vi "ValidateConfig.vi"(8 "error in (no error)":errorcluster, 11 "Channel in":refnum<class "Channel.lvclass">) -> (0 "error out":errorcluster, 2 "valid?":bool, 3 "Channel out":refnum<class "Channel.lvclass">)   [LabVIEW 2018, in "Channel.lvclass"]
uses:
  Channel.lvclass
  Channel.lvclass/Channel.ctl
  Interface/Interface.lvclass/Interface.ctl
  Interface/Interface.lvclass
panel:
  # "T=valid\nF=error"
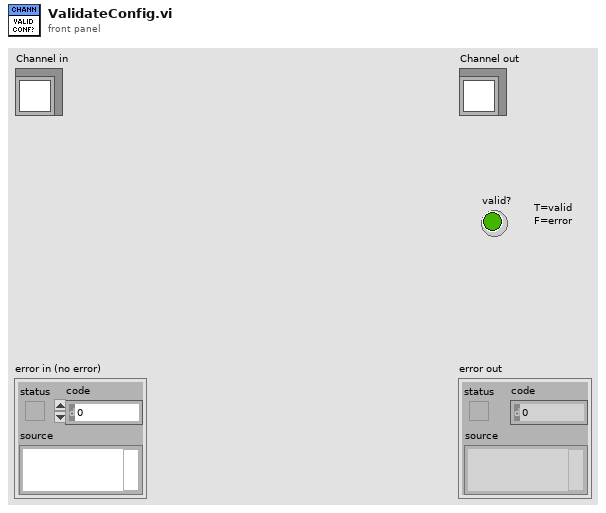
[diagram p1: front panel]
types:
  T1 = cluster{"ACQUISITION_MODE":u8, "TRIGGER_MODE":u8, "READ_MODE":u8, "PREAMP":u8, "READOUT_RATE":u8, "VERTICAL_SHIFT_SPEED":u8, "EM_MODE":u8, "EM_GAIN":u16, "SHUTTER_MODE":u8, "SHUTTER_TTL":u8, "SHUTTER_OPENING_TIME":u16, "SHUTTER_CLOSING_TIME":u16, "VBIN":u16, "HBIN":u16, "INITIAL_LINE":u16, "INITIAL_COLUMN":u16, "FINAL_LINE":u16, "FINAL_COLUMN":u16, "FRAME_TRANSFER":bool, "VERTICAL_CLOCK_VOLTAGE":u8, "AD_CHANNEL":u32}
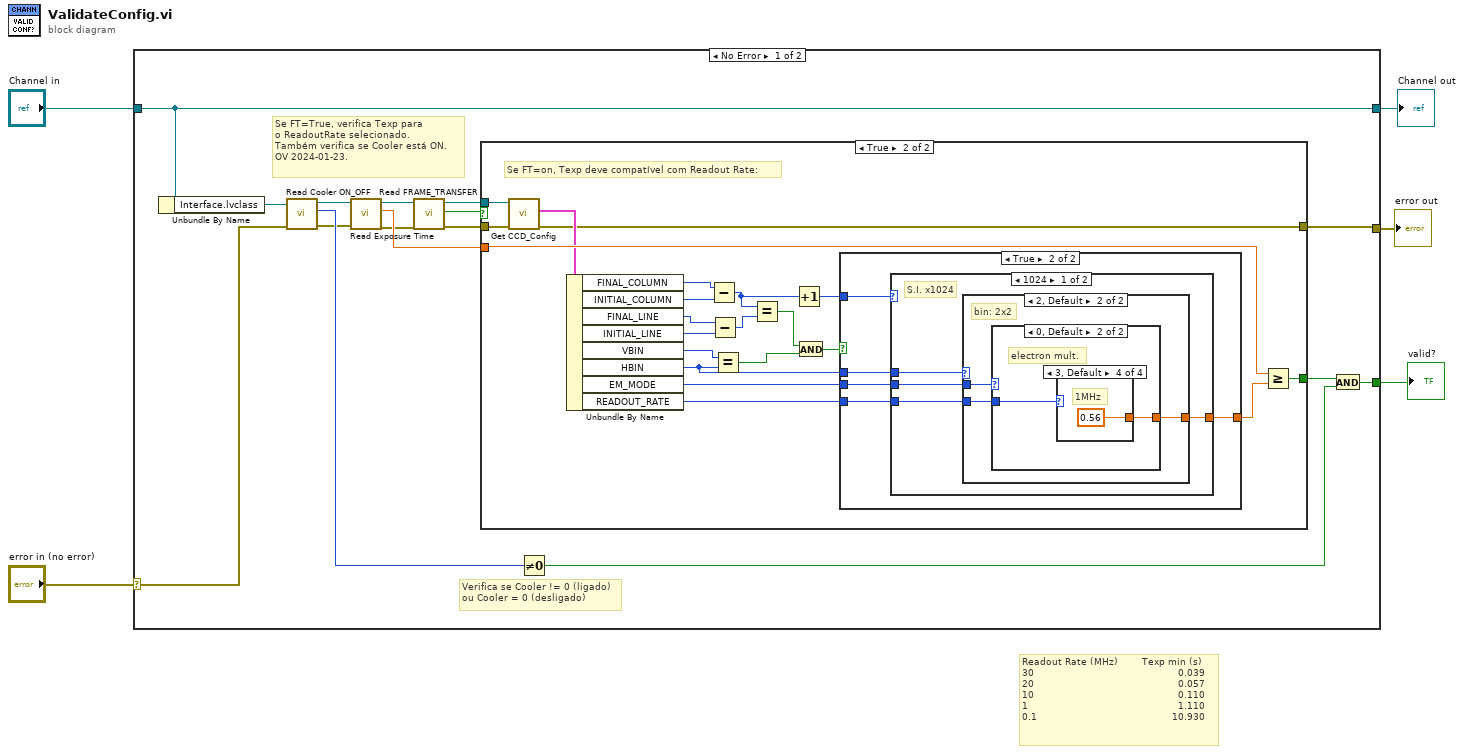
[diagram p0: block diagram]
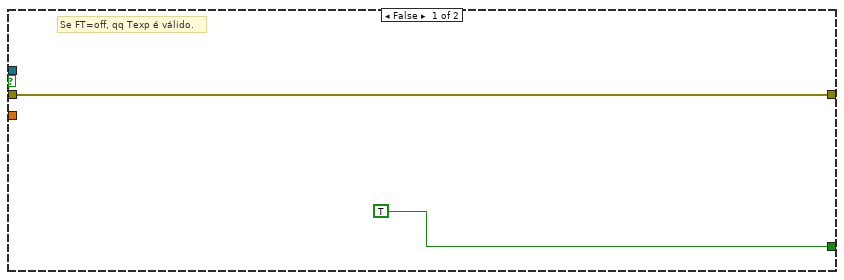
[diagram p2: hidden frame]
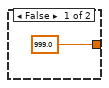
[diagram p3: hidden frame]
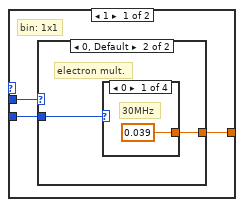
[diagram p4: hidden frame]
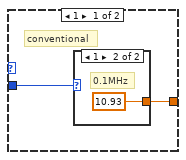
[diagram p5: hidden frame]
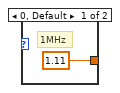
[diagram p6: hidden frame]
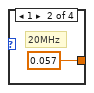
[diagram p7: hidden frame]
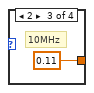
[diagram p8: hidden frame]
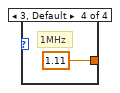
[diagram p9: hidden frame]
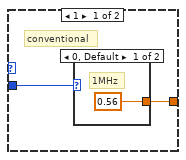
[diagram p10: hidden frame]
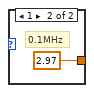
[diagram p11: hidden frame]
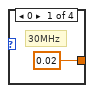
[diagram p12: hidden frame]
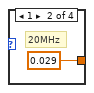
[diagram p13: hidden frame]
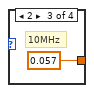
[diagram p14: hidden frame]
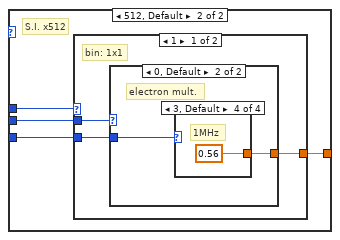
[diagram p15: hidden frame]
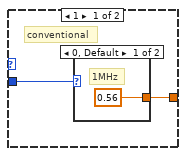
[diagram p16: hidden frame]
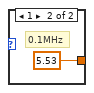
[diagram p17: hidden frame]
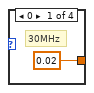
[diagram p18: hidden frame]
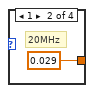
[diagram p19: hidden frame]
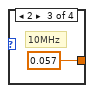
[diagram p20: hidden frame]
diagram:
  # "Readout Rate (MHz)        Texp min (s)\n30                                                0.039\n20                                                0.057  \n10                                                0.110\n1                                                  1.110\n0.1                                             10.930"
  n1 = case shown="No Error" "error in (no error)" {
    selector: "error in (no error)" -> [w14 w113]
    tunnel: [w6 w113] -> w4
    tunnel: [w21 w112] -> w2
    tunnel: "Channel in" -> [w21 w112]
    tunnel: [w11 FALSE] -> w1
    frame No Error {
      # "Verifica se Cooler != 0 (ligado)\nou Cooler = 0 (desligado)"
      # "Se FT=True, verifica Texp para \no ReadoutRate selecionado.\nTambém verifica se Cooler está ON.\nOV 2024-01-23."
      n2 = Unbundle By Name(w21) -> ("Interface.lvclass"=w17:refnum<class "Interface.lvclass">)
      n3 = call-dynamic "Read Cooler ON_OFF.vi"("error in (no error)"=w14, "Interface in"=w17) -> ("error out"=w13:errorcluster, "Cooler ON/OFF"=w15:i16, "Interface out"=w16:refnum<class "Interface.lvclass">)  [unwired: 7 in]
      n4 = call "Read Exposure Time.vi"("error in (no error)"=w13, "Interface in"=w16) -> ("error out"=w12:errorcluster, "Exposure Time"=w18:dbl, "Interface out"=w20:refnum<class "Interface.lvclass">)  [unwired: 7 in]
      n5 = call-dynamic "Read FRAME_TRANSFER.vi"("error in (no error)"=w12, "Interface in"=w20) -> ("error out"=w7:errorcluster, "FRAME_TRANSFER"=w19:bool, "Interface out"=w8:refnum<class "Interface.lvclass">)  [unwired: 7 in]
      n6 = case shown="True" w19 {
        tunnel: w18 -> [_ w44]
        tunnel: [TRUE w42] -> w10
        tunnel: w8 -> [_ w40]
        tunnel: w7 -> [w23 w39]
        tunnel: [w23 w36] -> w6
        frame False {
          # "Se FT=off, qq Texp é válido."
        }
        frame True {
          # "Se FT=on, Texp deve compatível com Readout Rate:"
          n7 = call-dynamic "Get CCD_Config.vi"("error in (no error)"=w39, "Interface in"=w40) -> ("error out"=w36:errorcluster, "output cluster"=w41:T1)  [unwired: 7 in, 1 out]
          n8 = Unbundle By Name(w41) -> ("FINAL_COLUMN"=w35:u16, "INITIAL_COLUMN"=w34:u16, "FINAL_LINE"=w33:u16, "INITIAL_LINE"=w32:u16, "VBIN"=w30:u16, "HBIN"=w25:u16, "EM_MODE"=w38:u8, "READOUT_RATE"=w37:u8)
          n9 = Subtract(x=w35, y=w34) -> (x-y=w26:u16)
          n10 = Subtract(x=w33, y=w32) -> (x-y=w31:u16)
          n11 = Equal?(x=w30, y=w25) -> (x = y?=w27:bool)
          n12 = Equal?(x=w26, y=w31) -> (x = y?=w28:bool)
          n13 = Increment(x=w26) -> (x+1=w24:u16)
          n14 = And(x=w28, y=w27) -> (x .and. y?=w29:bool)
          n15 = case shown="True" w29 {
            tunnel: [999.0 ("y") w50] -> w43
            tunnel: w38 -> [_ w49]
            tunnel: w37 -> [_ w48]
            tunnel: w24 -> [_ w47]
            tunnel: w25 -> [_ w46]
            frame False {
            }
            frame True {
              n16 = case shown="1024" w47 {
                tunnel: [w54 w84] -> w50
                tunnel: w49 -> [w53 w83]
                tunnel: w48 -> [w52 w82]
                tunnel: w46 -> [w51 w81]
                frame 1024 {
                  # "S.I. x1024"
                  n17 = case shown="2, Default" w51 {
                    tunnel: [w57 w70] -> w54
                    tunnel: w53 -> [w56 w69]
                    tunnel: w52 -> [w55 w68]
                    frame 1 {
                      # "bin: 1x1"
                      n18 = case shown="0, Default" w56 {
                        tunnel: [w59 w63] -> w57
                        tunnel: w55 -> [w58 w62]
                        frame 1 {
                          # "conventional"
                          n19 = case shown="1" w58 {
                            tunnel: [1.11 ("y") 10.93 ("y")] -> w59
                            frame 0, Default {
                              # "1MHz"
                            }
                            frame 1 {
                              # "0.1MHz"
                            }
                          }
                        }
                        frame 0, Default {
                          # "electron mult."
                          n20 = case shown="0" w62 {
                            tunnel: [0.039 ("y") 0.057 ("y") 0.11 ("y") 1.11 ("y")] -> w63
                            frame 0 {
                              # "30MHz"
                            }
                            frame 1 {
                              # "20MHz"
                            }
                            frame 2 {
                              # "10MHz"
                            }
                            frame 3, Default {
                              # "1MHz"
                            }
                          }
                        }
                      }
                    }
                    frame 2, Default {
                      # "bin: 2x2"
                      n21 = case shown="0, Default" w69 {
                        tunnel: [w72 w76] -> w70
                        tunnel: w68 -> [w71 w75]
                        frame 1 {
                          # "conventional"
                          n22 = case shown="0, Default" w71 {
                            tunnel: [0.56 ("y") 2.97 ("y")] -> w72
                            frame 0, Default {
                              # "1MHz"
                            }
                            frame 1 {
                              # "0.1MHz"
                            }
                          }
                        }
                        frame 0, Default {
                          # "electron mult."
                          n23 = case shown="3, Default" w75 {
                            tunnel: [0.02 ("y") 0.029 ("y") 0.057 ("y") 0.56 ("y")] -> w76
                            frame 0 {
                              # "30MHz"
                            }
                            frame 1 {
                              # "20MHz"
                            }
                            frame 2 {
                              # "10MHz"
                            }
                            frame 3, Default {
                              # "1MHz"
                            }
                          }
                        }
                      }
                    }
                  }
                }
                frame 512, Default {
                  # "S.I. x512"
                  n24 = case shown="1" w81 {
                    tunnel: [w87 w100] -> w84
                    tunnel: w83 -> [w86 w99]
                    tunnel: w82 -> [w85 w98]
                    frame 1 {
                      # "bin: 1x1"
                      n25 = case shown="0, Default" w86 {
                        tunnel: [w89 w93] -> w87
                        tunnel: w85 -> [w88 w92]
                        frame 1 {
                          # "conventional"
                          n26 = case shown="0, Default" w88 {
                            tunnel: [0.56 ("y") 5.53 ("y")] -> w89
                            frame 0, Default {
                              # "1MHz"
                            }
                            frame 1 {
                              # "0.1MHz"
                            }
                          }
                        }
                        frame 0, Default {
                          # "electron mult."
                          n27 = case shown="3, Default" w92 {
                            tunnel: [0.02 ("y") 0.029 ("y") 0.057 ("y") 0.56 ("y")] -> w93
                            frame 0 {
                              # "30MHz"
                            }
                            frame 1 {
                              # "20MHz"
                            }
                            frame 2 {
                              # "10MHz"
                            }
                            frame 3, Default {
                              # "1MHz"
                            }
                          }
                        }
                      }
                    }
                    frame 2, Default {
                      # "bin: 2x2"
                      n28 = case shown="0, Default" w99 {
                        tunnel: [w102 w106] -> w100
                        tunnel: w98 -> [w101 w105]
                        frame 1 {
                          # "conventional"
                          n29 = case shown="0, Default" w101 {
                            tunnel: [0.28 ("y") 2.14 ("y")] -> w102
                            frame 0, Default {
                              # "1MHz"
                            }
                            frame 1 {
                              # "0.1MHz"
                            }
                          }
                        }
                        frame 0, Default {
                          # "electron mult."
                          n30 = case shown="3, Default" w105 {
                            tunnel: [0.011 ("y") 0.015 ("y") 0.029 ("y") 0.28 ("y")] -> w106
                            frame 0 {
                              # "30MHz"
                            }
                            frame 1 {
                              # "20MHz"
                            }
                            frame 2 {
                              # "10MHz"
                            }
                            frame 3, Default {
                              # "1MHz"
                            }
                          }
                        }
                      }
                    }
                  }
                }
              }
            }
          }
          n31 = Greater Or Equal?(x=w44, y=w43) -> (x >= y?=w42:bool)
        }
      }
      n32 = Not Equal To 0?(x=w15) -> (x != 0?=w9:bool)
      n33 = And(x=w10, y=w9) -> (x .and. y?=w11:bool)
    }
    frame Error {
    }
  }
  "error out" <- w4
  "Channel out" <- w2
  "valid?" <- w1
